vi "ProcesadorDTMFSignalsV2.vi"() -> ()   [LabVIEW 2020]
uses:
  <vilib>/measure/matone.llb/Extract Multiple Tone Information N Chan.vi
  <vilib>/measure/matone.llb/Extract Multiple Tone Information 1 Chan.vi
  <vilib>/express/express analysis/Spectral/Block/exnSpectralBlock spectral measurements peak poly.vi
  <vilib>/express/express analysis/Spectral/Block/exnSpectralBlock spectral measurements peak DDT.vi
  <vilib>/express/express analysis/Spectral/XNode/ExpressSpectralMeasurementsBlockNode.xnode
  <vilib>/measure/NI_MAPro.lvlib
panel:
  out "Max_frequency 2":dbl
  out "Min_frequency 2":dbl
  out "Max_frequency":dbl
  out "Min_frequency":dbl
  out "Waveform Graph":dynamicdata(graph)=[{"t0"=timestamp(0 s since 1904-01-01), "dt"=2.0001814223512335, "Y"=array[5512 elements], "attributes"=variant("NI_ChannelName"=variant(string "FFT - (Peak)"))}, {"t0"=timestamp(0 s since 1904-01-01), "dt"=2.0001814223512335, "Y"=array[5512 elements], "attributes"=variant("NI_ChannelName"=variant(string "FFT - (Peak)"))}]
  in  "stop":bool
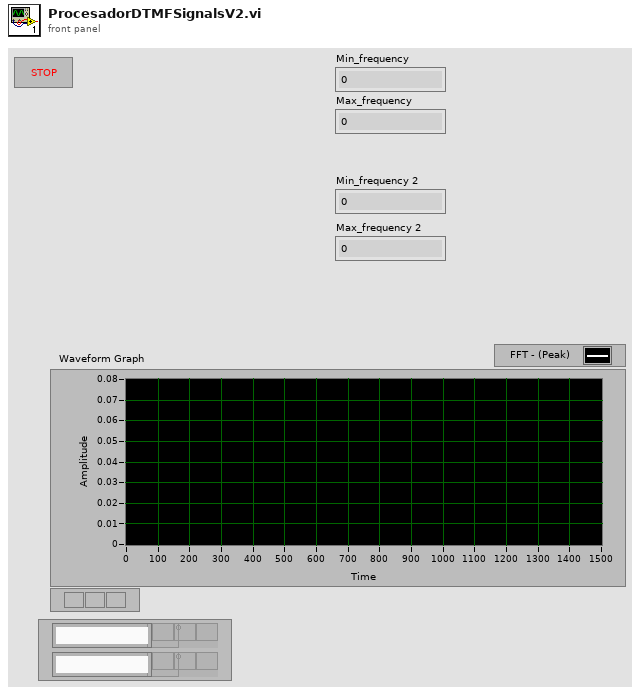
[diagram p1: front panel]
types:
  T1 = cluster{"averaging mode":u16, "weighting mode":u16, "number of averages":u32}
  T2 = cluster{"dB On (F)":bool, "unwrap phase (F)":bool, "convert to degree (F)":bool}
  T3 = cluster{"multiple tone information":cluster{"detected frequency":dbl, "detected amplitude":dbl, "detected phase (deg)":dbl}[]}[]
  T4 = cluster{"multiple tone information":cluster{"detected frequency":dbl, "detected amplitude":dbl, "detected phase (deg)":dbl}[]}
  T5 = cluster{"detected frequency":dbl, "detected amplitude":dbl, "detected phase (deg)":dbl}[]
  T6 = cluster{"detected frequency":dbl, "detected amplitude":dbl, "detected phase (deg)":dbl}
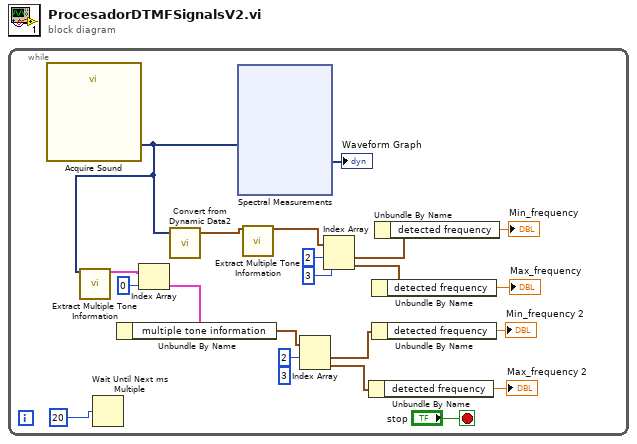
[diagram p0: block diagram]
diagram:
  n1 = while {
    stop <- "stop" stop-if-true
    (unwired) 3 ("index")
    n2 = call "Acquire Sound"() -> ("Data"=w10:dynamicdata)  [unwired: 18 in, 1 out]
    n3 = call-poly <vilib>:"Extract Multiple Tone Information.vi"("time signals in"=w10) -> ("multiple tone information"=w9:T3)  [unwired: 12 in, 2 out]
    n4 = Wait Until Next ms Multiple(millisecond multiple=u32 20) -> ()  [unwired: 1 out]
    n5 = Index Array(array=w9, index=0) -> (element=w7:T4)
    n6 = Unbundle By Name(w7) -> ("multiple tone information"=w5:T5)
    n7 = call "Convert from Dynamic Data2"("Dynamic Data Type"=w10) -> ("Waveform"=w20:waveform(dbl))  [unwired: 3 in]
    n8 = xnode "Spectral Measurements"("Signals"=w10) -> ("FFT - (Peak)"=→"Waveform Graph":dynamicdata)  [unwired: 1 in, 2 out]
    n9 = call-poly <vilib>:"Extract Multiple Tone Information.vi"("time signal in"=w20) -> ("multiple tone information"=w19:T5)  [unwired: 12 in, 2 out]
    n10 = Index Array(array=w5, index #1=2 ("index")) -> (element #1=w2:T6, element #2=w1:T6)  [unwired: 1 in]
    n11 = Index Array(array=w19, index #1=2 ("index"), index #2=3 ("index")) -> (element #1=w15:T6, element #2=w14:T6)
    n12 = Unbundle By Name(w1) -> ("detected frequency"=→"Max_frequency 2":dbl)
    n13 = Unbundle By Name(w14) -> ("detected frequency"=→"Max_frequency":dbl)
    n14 = Unbundle By Name(w2) -> ("detected frequency"=→"Min_frequency 2":dbl)
    n15 = Unbundle By Name(w15) -> ("detected frequency"=→"Min_frequency":dbl)
  }
